vi "Configure Output Trigger.vi"(0 "VISA resource name":refnum<visa-resource-name>, 1 "Enable Trigger Output (F: Disable)":bool, 2 "Internal Trigger Line (1: Line 1)":i32(ring)=1 items=["Line 1"=1, "Line 2"=2], 5 "Channel (1: Channel 1)":i32(ring)=1 items=["Channel 1"=1, "Channel 2"=2], 7 "Trigger Location (0: Idle-ARM)":i32(ring) items=["Idle-ARM", "ARM-Trigger", "Trigger-Acquire", "Trigger-Transient"], 9 "Trigger Signal (1: EXT1)":i32(ring)=1 items=["EXT1"=1, "EXT2"=2, "EXT3"=3, "EXT4"=4, "EXT5"=5, "EXT6"=6, "EXT7"=7, "LAN"=8, "Internal Bus 1"=9, "Internal Bus 2"=10], 11 "error in (no error)":errorcluster, 12 "Device Action (2: Both)":i32(ring)=2 items=["Acquire", "Transient", "Both"], 13 "Trigger Timing (2: Both)":i32(ring)=2 items=["Before", "After", "Both"]) -> (4 "VISA resource name out":refnum<visa-resource-name>, 15 "error out":errorcluster)   [LabVIEW 2012, in "Keysight B2980 Series.lvlib"]
doc: "Configures output triggers for status change between idle-arm, arm-trigger or trigger-action layer.\n\n<b>Note(s):</b>\nThis VI is only applicable for model B2985A and B2987A."
uses:
  Keysight B2980 Series.lvlib
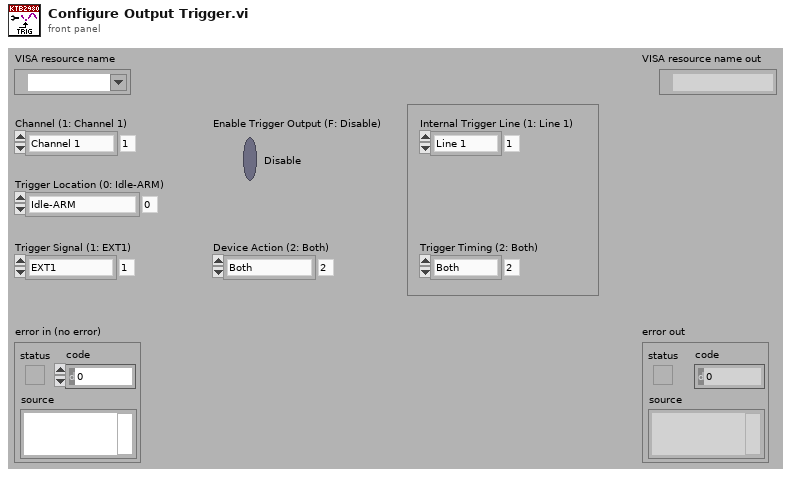
[diagram p1: front panel]
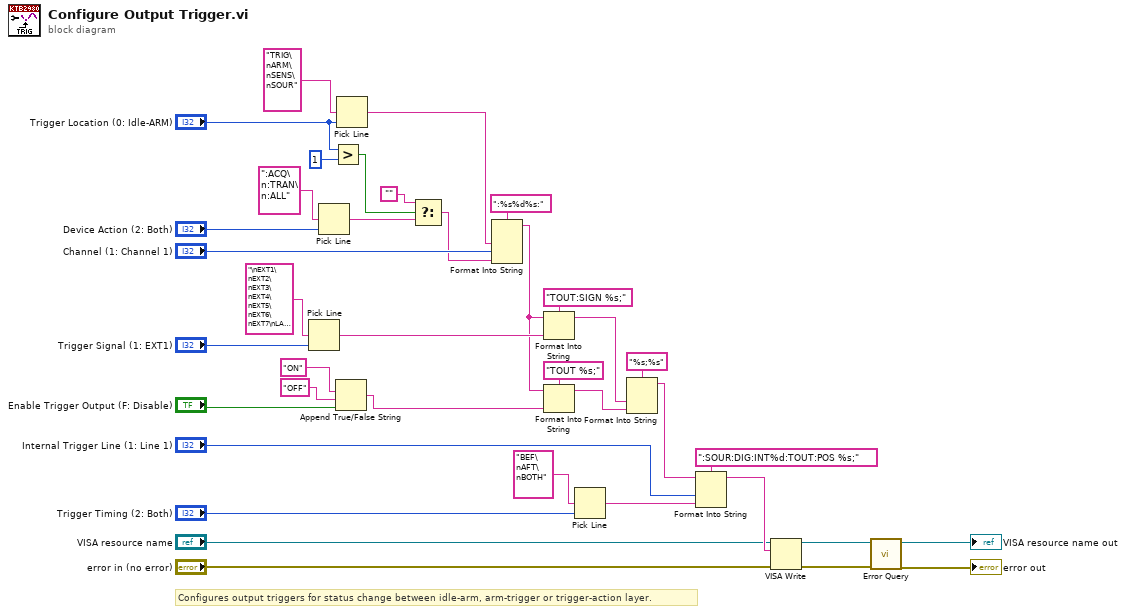
[diagram p0: block diagram]
diagram:
  # "Configures output triggers for status change between idle-arm, arm-trigger or trigger-action layer."
  n1 = Pick Line(multi-line string="\nEXT1\nEXT2\nEXT3\nEXT4\nEXT5\nEXT6\nEXT7\nLAN\nINT1\nINT2", line index="Trigger Signal (1: EXT1)") -> (output string=w8:string)  [unwired: 1 out]
  n2 = Pick Line(multi-line string=":ACQ\n:TRAN\n:ALL", line index="Device Action (2: Both)") -> (output string=w17:string)  [unwired: 1 out]
  n3 = Greater?(x="Trigger Location (0: Idle-ARM)", y=1) -> (0:w16:bool)
  n4 = Append True/False String(1:"Enable Trigger Output (F: Disable)", 2:"OFF", 3:"ON") -> (0:w5:string)  [unwired: 1 out]
  n5 = Pick Line(multi-line string="TRIG\nARM\nSENS\nSOUR", line index="Trigger Location (0: Idle-ARM)") -> (output string=w13:string)  [unwired: 1 out]
  n6 = Select(t="", s=w16, f=w17) -> (s? t:f=w11:string)
  n7 = Format Into String(format string=":%s%d%s:", w13, "Channel (1: Channel 1)", w11) -> (resulting string=w6:string)  [unwired: 2 in, 1 out]
  n8 = Format Into String(format string="TOUT:SIGN %s;", initial string=w6, w8) -> (resulting string=w3:string)  [unwired: 1 in, 1 out]
  n9 = Format Into String(format string="TOUT %s;", initial string=w6, w5) -> (resulting string=w2:string)  [unwired: 1 in, 1 out]
  n10 = Pick Line(multi-line string="BEF\nAFT\nBOTH", line index="Trigger Timing (2: Both)") -> (output string=w28:string)  [unwired: 1 out]
  n11 = Format Into String(format string="%s;%s", w3, w2) -> (resulting string=w1:string)  [unwired: 2 in, 1 out]
  n12 = Format Into String(format string=":SOUR:DIG:INT%d:TOUT:POS %s;", initial string=w1, "Internal Trigger Line (1: Line 1)", w28) -> (resulting string=w27:string)  [unwired: 1 in, 1 out]
  n13 = VISA Write(VISA resource name="VISA resource name", write buffer=w27, error in (no error)="error in (no error)") -> (VISA resource name out=w24:refnum<visa-resource-name>, error out=w23:errorcluster)  [unwired: 1 out]
  n14 = call "Error Query.vi"("error in (no error)"=w23, "VISA resource name"=w24) -> ("error out"=→"error out":errorcluster, "VISA resource name out"=→"VISA resource name out":refnum<visa-resource-name>)  [unwired: 8 out]
